vi "Vision-Ball.vi"(10 "Minimum Confidence":dbl=0.15) -> (0 "Confidence":dbl, 1 "z Coordinate of Ball":dbl, 2 "y Coordinate of Ball":dbl, 3 "x Coordinate of Ball":dbl, 5 "ball detected":bool)   [LabVIEW 2015]
uses:
  <vilib>/Analysis/Matrix/Datatypes/RealMatrix.ctl
  labview-zmq/socket_type.ctl
  labview-zmq/socket_options.ctl
  <vilib>/Analysis/Matrix/Numeric/Conversions/Array To Matrix - RA2.vi
  labview-zmq/zmq_socket.lvclass
  labview-zmq/zeromq.lvlib
  labview-zmq/zmq_context.lvclass
  <vilib>/Rock Robotics/Network Tables/NT Read Number.vi
  <vilib>/Analysis/Matrix/NI_Matrix.lvlib
panel:
  in  "Reset":bool
  out "Real Matrix":T1
  in  "Max height":dbl
  out "data":string
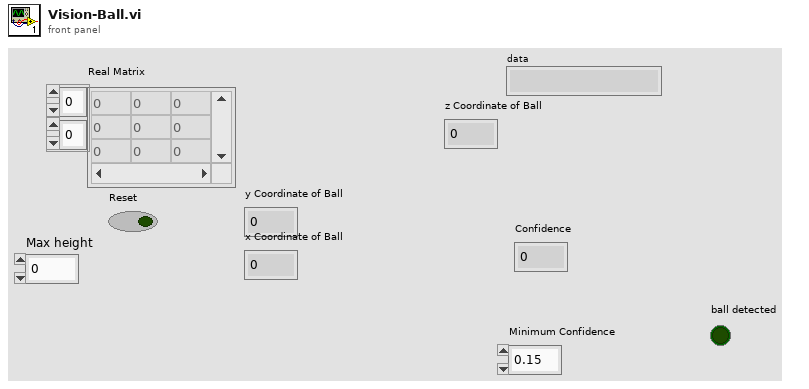
[diagram p1: front panel]
types:
  T1 = typedef "NI_Matrix.lvlib/RealMatrix.ctl" = dbl[][]
  T2 = typedef "zeromq.lvlib/socket_options.ctl" = enum8{"NONE", "ZMQ_HWM", "<2>", "ZMQ_SWAP", "ZMQ_AFFINITY", "ZMQ_IDENTITY", "ZMQ_SUBSCRIBE", "ZMQ_UNSUBSCRIBE", "ZMQ_RATE", "ZMQ_RECOVERY_IVL", "ZMQ_MCAST_LOOP", "ZMQ_SNDBUF", "ZMQ_RCVBUF", "ZMQ_RCVMORE", "ZMQ_FD", "ZMQ_EVENTS", "ZMQ_TYPE", "ZMQ_LINGER", "ZMQ_RECONNECT_IVL", "ZMQ_BACKLOG", "ZMQ_RECOVERY_IVL_MSEC", "ZMQ_RECONNECT_IVL_MAX", "ZMQ_MAXMSGSIZE", "ZMQ_SNDHWM", "ZMQ_RCVHWM", "ZMQ_MULTICAST_HOPS", "<26>", "ZMQ_RCVTIMEO", "ZMQ_SNDTIMEO", "<29>", "<30>", "ZMQ_IPV4ONLY", "ZMQ_LAST_ENDPOINT", "ZMQ_ROUTER_MANDATORY", "ZMQ_TCP_KEEPALIVE", "ZMQ_TCP_KEEPALIVE_CNT", "ZMQ_TCP_KEEPALIVE_IDLE", "ZMQ_TCP_KEEPALIVE_INTVL", "ZMQ_TCP_ACCEPT_FILTER", "ZMQ_DELAY_ATTACH_ON_CONNECT", "ZMQ_XPUB_VERBOSE"}
  T3 = typedef "zeromq.lvlib/socket_type.ctl" = enum8{"ZMQ_PAIR", "ZMQ_PUB", "ZMQ_SUB", "ZMQ_REQ", "ZMQ_REP", "ZMQ_DEALER", "ZMQ_ROUTER", "ZMQ_PULL", "ZMQ_PUSH", "ZMQ_XPUB", "ZMQ_XSUB"}
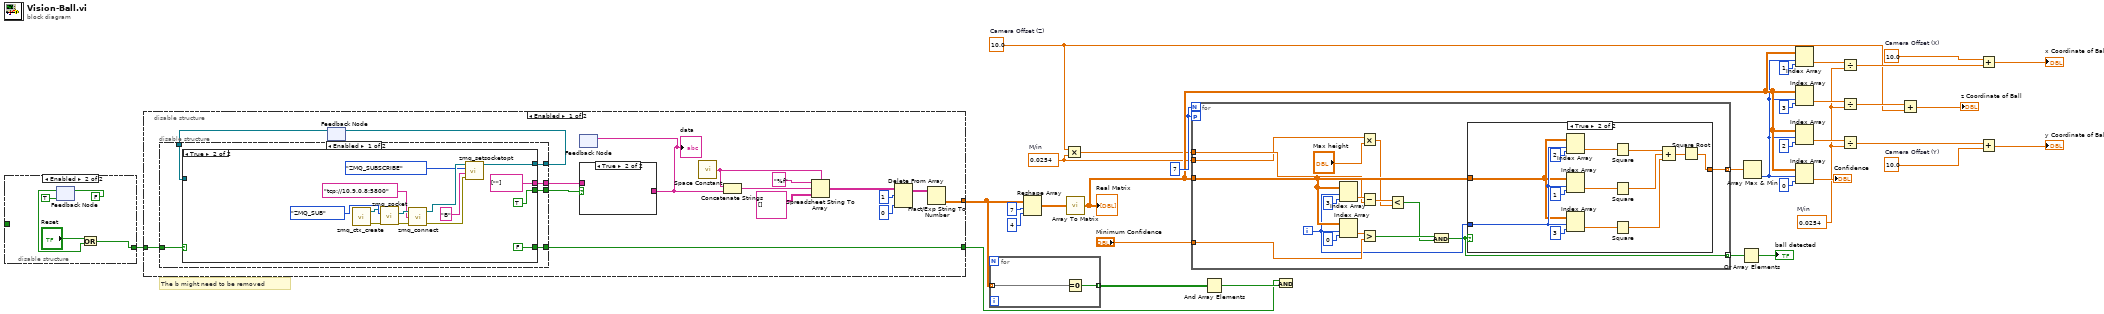
[diagram p0: block diagram]
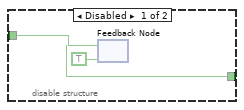
[diagram p2: hidden frame]
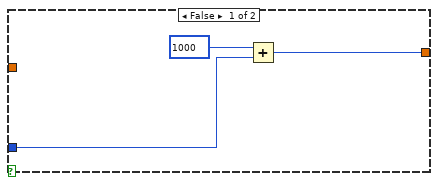
[diagram p3: hidden frame]
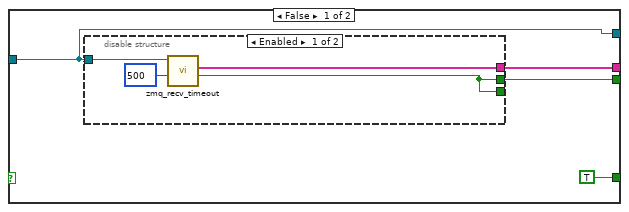
[diagram p4: hidden frame]
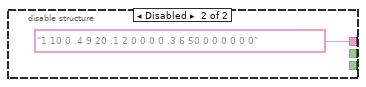
[diagram p5: hidden frame]
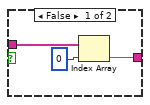
[diagram p7: hidden frame]
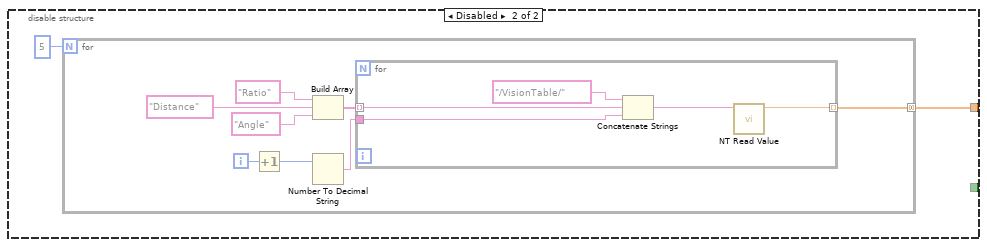
[diagram p8: hidden frame]
diagram:
  w5 = 0.0254  # M/in
  w8 = 0.0254  # M/in
  w4 = 10.0  # Camera Offset (Y)
  w3 = 10.0  # Camera Offset (X)
  w7 = 10.0  # Camera Offset (Z)
  w32 = 7
  # "The b might need to be removed"
  n1 = disable-structure shown="Enabled" {
    disable-tunnel: _ -> [w38 _]
    disable-tunnel: [w36 w41] -> w1
    frame Disabled {
      n2 = feedback #1(TRUE) -> (w36:bool)
      n3 = feedback-in #1(w38) -> ()
    }
    frame Enabled {
      n4 = feedback-in #2(FALSE) -> ()
      n5 = feedback #2(TRUE) -> (w40:bool)
      n6 = Or(x="Reset", y=w40) -> (x .or. y?=w41:bool)
    }
  }
  n7 = disable-structure shown="Enabled" {
    disable-tunnel: [w53 w93] -> w2
    disable-tunnel: w1 -> [w44 _]
    disable-tunnel: [w45 _] -> w22
    frame Enabled {
      n8 = feedback #3() -> (w46:refnum<class "zmq_socket.lvclass">)  [unwired: 1 in]
      n9 = disable-structure shown="Enabled" {
        disable-tunnel: [w65 _] -> w49
        disable-tunnel: [w64 _] -> w48
        disable-tunnel: [w63 _] -> w47
        disable-tunnel: w46 -> [w62 _]
        disable-tunnel: [w61 _] -> w45
        disable-tunnel: w44 -> [w60 _]
        frame Enabled {
          n10 = case shown="True" w60 {
            tunnel: [w69 string[] [""] ("parts")] -> w65
            tunnel: [w68 TRUE ("timeout?")] -> w64
            tunnel: w62 -> [w67 _]
            tunnel: [w67 w77] -> w63
            tunnel: [TRUE FALSE] -> w61
            frame False {
              n11 = disable-structure shown="Enabled" {
                disable-tunnel: [w73 "1 10 0 .4 9 20 .1 2 0 0 0 0 .3 6 50 0 0 0 0 0 0"] -> w69
                disable-tunnel: [w71 _] -> w68
                disable-tunnel: [w71 _] -> _
                disable-tunnel: w67 -> [w70 _]
                frame Enabled {
                  n12 = call "zmq_recv_timeout.vi"("timeout (ms)"=u32 500, "socket in"=w70) -> ("timeout?"=w71:bool, "parts"=w73:string[])  [unwired: 2 in, 2 out]
                }
                frame Disabled {
                }
              }
            }
            frame True {
              n13 = call "zmq_ctx_create.vi"() -> ("error out"=w84:errorcluster, "context out"=w87:refnum<class "zmq_context.lvclass">)  [unwired: 4 in]
              n14 = call "zmq_socket.vi"("error in"=w84, "socket type"=socket_type."ZMQ_SUB", "context in"=w87) -> ("error out"=w81:errorcluster, "socket out"=w86:refnum<class "zmq_socket.lvclass">)  [unwired: 2 in, 1 out]
              n15 = call "zmq_connect.vi"("error in"=w81, "endpoint"="tcp://10.9.0.8:5800" ("Endpoint"), "socket in"=w86) -> ("error out"=w82:errorcluster, "socket out"=w83:refnum<class "zmq_socket.lvclass">)  [unwired: 1 in]
              n16 = call "zmq_setsocketopt.vi"("error in"=w82, "value"="B", "option"=socket_options."ZMQ_SUBSCRIBE", "socket in"=w83) -> ("socket out"=w77:refnum<class "zmq_socket.lvclass">)  [unwired: 2 in, 1 out]
            }
          }
        }
        frame Disabled {
        }
      }
      n17 = feedback-in #3(w47) -> ()
      n18 = feedback #4() -> ()  [unwired: 2 in]
      n19 = case shown="True" w48 {
        tunnel: w49 -> [w91 _]
        tunnel: [w89 _] -> w50
        frame False {
          n20 = Index Array(array=w91, index=0) -> (element=w89:string)
        }
        frame True {
        }
      }
      "data" <- w50
      n21 = feedback-in #4(w50) -> ()
      n22 = call <vilib>:"Space Constant.vi"() -> ("String"=w51:string)
      n23 = Concatenate Strings(w51, w50) -> (w52:string)
      n24 = Spreadsheet String To Array(delimiter (Tab)=w51, format string="%f", spreadsheet string=w52, array type (2D Dbl)=string[][] [] ("Array")) -> (array=w54:string[][])
      n25 = Delete From Array(array=w54, length=1, index (col)=0 ("disabled index (col)")) -> (array with subset deleted=w55:string[][])  [unwired: 1 in, 1 out]
      n26 = Fract/Exp String To Number(string=w55) -> (number=w53:dbl[][])  [unwired: 4 out]
    }
    frame Disabled {
      n27 = for {
        N: 5 -> [_]
        tunnel: [w101] -> w93 mode=concatenating
        i -> [w96]
        n28 = Increment(x=w96) -> (x+1=w95:i32)
        n29 = Build Array("Ratio" ("element"), "Distance" ("element"), "Angle") -> (w97:string[])
        n30 = Number To Decimal String(number=w95) -> (decimal integer string=w94:string)  [unwired: 1 in]
        n31 = for {
          tunnel: [w105] -> w101 mode=indexing
          tunnel: w97 -> [w104] mode=indexing
          tunnel: w94 -> [w102]
          n32 = Concatenate Strings("/VisionTable/" ("string"), w104, w102) -> (w106:string)
          n33 = call-poly <vilib>:"NT Read Value.vi"("Name"=w106) -> ("Numeric"=w105:dbl)  [unwired: 9 in, 1 out]
        }
      }
    }
  }
  n34 = for {
    tunnel: w2 -> [w108] mode=indexing
    tunnel: [w107] -> w24 mode=indexing
    n35 = Equal To 0?(x=w108) -> (x = 0?=w107:bool[])
  }
  n36 = Reshape Array(w2, 7 ("dimension size"), 4 ("dimension size")) -> (w33:dbl[][])
  n37 = Multiply(x=w7, y=w5) -> (x*y=w6:dbl)
  n38 = call-poly <vilib>:"Array To Matrix.vi"("Real 2D Array"=w33) -> ("Real Matrix"=w20:T1)
  "Real Matrix" <- w20
  n39 = for {
    N: w32 -> [_]
    workers-P: w32 -> [_]
    tunnel: w20 -> [w119]
    tunnel: "Minimum Confidence" -> [w123]
    tunnel: [w121] -> w30 mode=indexing
    tunnel: [w111] -> w12 mode=indexing
    tunnel: w6 -> [w115]
    tunnel: w5 -> [w109]
    i -> [w118]
    n40 = Index Array(array=w119, index (row)=w118, index (col)=3) -> (element=w117:dbl)
    n41 = Index Array(array=w119, index (row)=w118, index (col)=0) -> (element=w124:dbl)
    n42 = Multiply(x=w109, y="Max height") -> (x*y=w110:dbl)
    n43 = Subtract(x=w117, y=w115) -> (x-y=w116:dbl)
    n44 = Greater?(x=w124, y=w123) -> (0:w113:bool)
    n45 = Less?(x=w116, y=w110) -> (x < y?=w112:bool)
    n46 = And(x=w113, y=w112) -> (x .and. y?=w111:bool)
    n47 = case shown="True" w111 {
      tunnel: w118 -> [w125 w137]
      tunnel: w119 -> [_ w136]
      tunnel: [w126 w128] -> w121
      frame False {
        n48 = Add(x=1000, y=w125) -> (x+y=w126:i32)
      }
      frame True {
        n49 = Index Array(array=w136, index (row)=w137, index (col)=2) -> (element=w135:dbl)
        n50 = Index Array(array=w136, index (row)=w137, index (col)=1) -> (element=w133:dbl)
        n51 = Index Array(array=w136, index (row)=w137, index (col)=3) -> (element=w134:dbl)
        n52 = Square(x=w135) -> (x^2=w132:dbl)
        n53 = Square(x=w133) -> (x^2=w131:dbl)
        n54 = Square(x=w134) -> (x^2=w130:dbl)
        n55 = Compound Arithmetic op=ADD(w132, w131, w130) -> (w129:dbl)
        n56 = Square Root(x=w129) -> (sqrt(x)=w128:dbl)
      }
    }
  }
  n57 = And Array Elements(Boolean array=w24) -> (logical AND=w23:bool)
  n58 = And(x=w22, y=w23) -> ()  [unwired: 1 out]
  n59 = Or Array Elements(Boolean array=w12) -> (logical OR=→"ball detected":bool)
  n60 = Array Max & Min(array=w30) -> (min index (indices)=w19:i32)  [unwired: 3 out]
  n61 = Index Array(array=w20, index (row)=w19, index (col)=1) -> (element=w18:dbl)
  n62 = Index Array(array=w20, index (row)=w19, index (col)=3) -> (element=w16:dbl)
  n63 = Index Array(array=w20, index (row)=w19, index (col)=2) -> (element=w17:dbl)
  n64 = Index Array(array=w20, index (row)=w19, index (col)=0) -> (element=→"Confidence":dbl)
  n65 = Divide(x=w18, y=w8) -> (x/y=w10:dbl)
  n66 = Divide(x=w16, y=w8) -> (x/y=w9:dbl)
  n67 = Divide(x=w17, y=w8) -> (x/y=w11:dbl)
  n68 = Add(x=w9, y=w7) -> (x+y=→"z Coordinate of Ball":dbl)
  n69 = Add(x=w3, y=w10) -> (x+y=→"x Coordinate of Ball":dbl)
  n70 = Add(x=w11, y=w4) -> (x+y=→"y Coordinate of Ball":dbl)
